vi "Parallel Execution A.vi"() -> (0 "error out A":errorcluster)   [LabVIEW 2020]
panel:
  out "Iterations A":i32
  in  "Write Value A":dbl=1.5 format="%.6f"
  in  "Write Name A":string="DAC0"
  in  "stop":bool
  out "Error String A":string
  out "Read Value A":dbl format="%.6f"
  in  "Read Name A":string="AIN0"
  out "ConnectionType Out":i32
  out "DeviceType Out":i32
  in  "Identifier":string="470013239"
  in  "ConnectionType":string="usb"
  in  "DeviceType":string="t7"
  # "Open and run these A and B examples at the same time to demonstrate 2 parallel VIs talking to the same device.  See more related\ncomments on the block diagram of \"Parallel Execution.vi\", but the main reasons this works:\n\n1.  Neither VI is calling Close.\n2.  Both VIs are in the same thread.\n\nWe recommend opening with specific values here rather than using any-any-any to search for a device.  Since both VIs (A and B) will\nmake an open call we want to make sure they both open the same device."
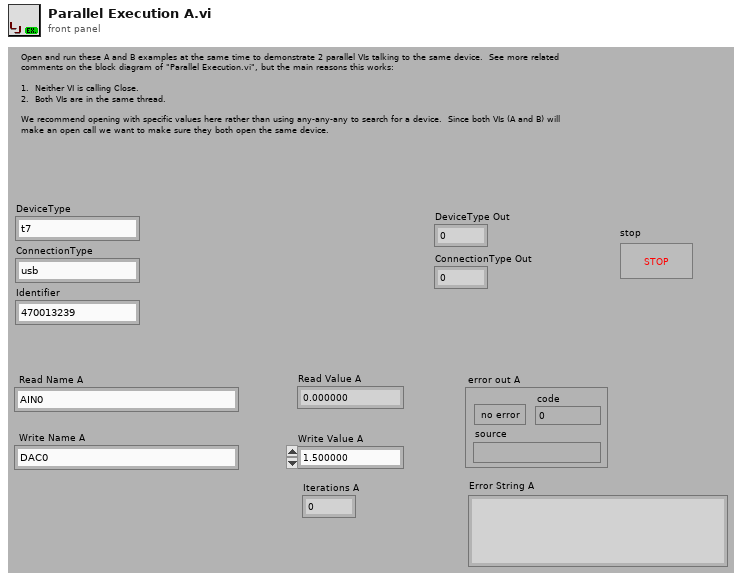
[diagram p1: front panel]
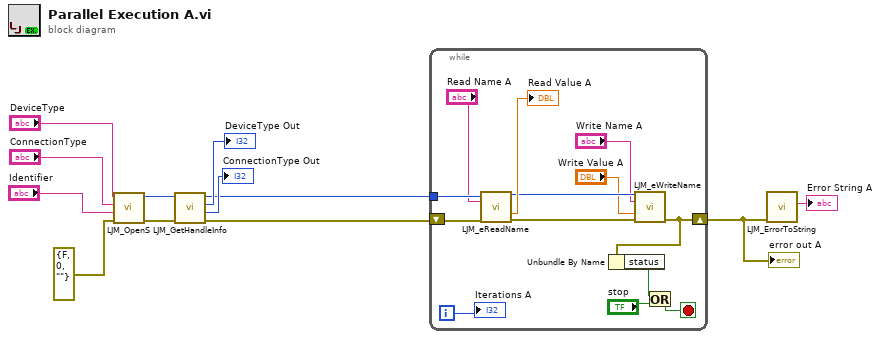
[diagram p0: block diagram]
diagram:
  n1 = call "LJM_OpenS.vi"("error in"=errorcluster {"status"=FALSE, "code"=0, "source"=""} ("error in (no error)"), "Identifier"="Identifier", "ConnectionType"="ConnectionType", "DeviceType"="DeviceType") -> ("error out"=w11:errorcluster, "Handle"=w10:i32)  [unwired: 6 in]
  n2 = call "LJM_GetHandleInfo.vi"("error in"=w11, "Handle In"=w10) -> ("error out"=w1:errorcluster, "ConnectionType"=→"ConnectionType Out":i32, "DeviceType"=→"DeviceType Out":i32, "Handle Out"=w2:i32)  [unwired: 2 in, 4 out]
  n3 = while {
    tunnel: w2 -> [w24]
    shift-right: [w17] -> w3
    shift-left: w1 -> [w25]
    i -> [w13]
    stop <- w21 stop-if-true
    n4 = call "LJM_eReadName.vi"("Handle In"=w24, "Name"="Read Name A", "error in"=w25) -> ("Handle Out"=w16:i32, "Value"=→"Read Value A":dbl, "error out"=w18:errorcluster)  [unwired: 10 in]
    n5 = call "LJM_eWriteName.vi"("Handle In"=w16, "Name"="Write Name A", "Value"="Write Value A", "error in"=w18) -> ("error out"=w17:errorcluster)  [unwired: 10 in, 1 out]
    n6 = Unbundle By Name(w17) -> ("status"=w19:bool)
    n7 = Or(x=w19, y="stop") -> (x .or. y?=w21:bool)
    "Iterations A" <- w13
  }
  "error out A" <- w3
  n8 = call "LJM_ErrorToString.vi"("error in"=w3) -> ("String"=→"Error String A":string)  [unwired: 10 in]
